vi "Format Resistor.vi"(3 "Resistor Value":dbl format="%#.3f") -> (0 "Band 2":dbl, 1 "Band 1":dbl, 2 "Band3":dbl)   [LabVIEW 2014]
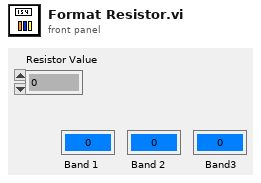
[diagram p1: front panel]
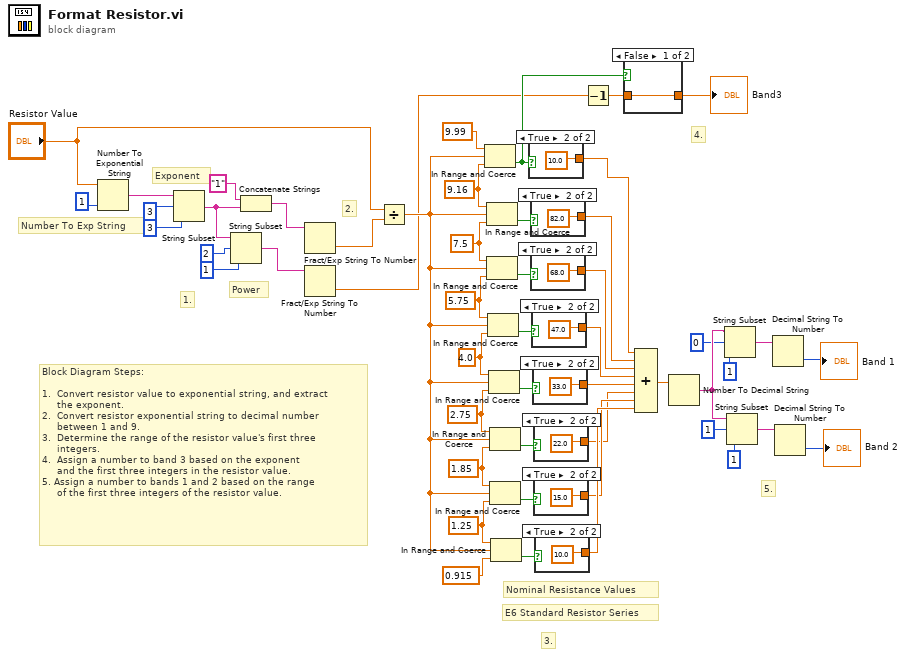
[diagram p0: block diagram]
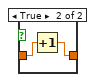
[diagram p2: hidden frame]
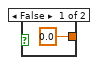
[diagram p3: hidden frame]
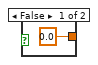
[diagram p4: hidden frame]
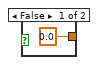
[diagram p5: hidden frame]
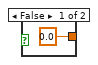
[diagram p6: hidden frame]
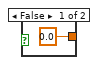
[diagram p7: hidden frame]
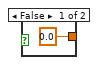
[diagram p8: hidden frame]
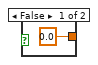
[diagram p9: hidden frame]
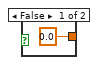
[diagram p10: hidden frame]
diagram:
  w21 = 9.16
  w27 = 7.5
  w29 = 5.75
  w26 = 4.0
  w35 = 2.75
  w34 = 1.85
  w40 = 1.25
  # "E6 Standard Resistor Series"
  # "Block Diagram Steps:\n\n1.  Convert resistor value to exponential string, and extract\n     the exponent.\n2.  Convert resistor exponential string to decimal number \n     between 1 and 9.\n3.  Determine the range of the resistor value's first three\n     integers.\n4.  Assign a number to band 3 based on the exponent\n     and the first three integers in the resistor value.\n5. Assign a number to bands 1 and 2 based on the range\n     of the first three integers of the resistor value."
  # "5."
  # "4."
  # "3."
  # "2."
  # "1."
  # "Power"
  # "Exponent"
  # "Number To Exp String"
  # "Nominal Resistance Values"
  n1 = Number To Exponential String(number="Resistor Value", precision (6)=i16 1) -> (E-format string=w49:string)  [unwired: 2 in]
  n2 = String Subset(string=w49, offset (0)=3, length (rest)=3 ("length (rest)")) -> (substring=w18:string)
  n3 = String Subset(string=w18, offset (0)=2, length (rest)=1 ("length (rest)")) -> (substring=w16:string)
  n4 = Concatenate Strings("1" ("string"), w18) -> (w45:string)
  n5 = Fract/Exp String To Number(string=w45) -> (number=w46:dbl)  [unwired: 3 in, 1 out]
  n6 = Fract/Exp String To Number(string=w16) -> (number=w12:dbl)  [unwired: 3 in, 1 out]
  n7 = Divide(x="Resistor Value", y=w46) -> (x/y=w15:dbl)
  n8 = In Range and Coerce(upper limit=9.99, x=w15, lower limit=w21) -> (In Range?=w14:bool)  [unwired: 1 out]
  n9 = In Range and Coerce(upper limit=w21, x=w15, lower limit=w27) -> (In Range?=w28:bool)  [unwired: 1 out]
  n10 = In Range and Coerce(upper limit=w27, x=w15, lower limit=w29) -> (In Range?=w30:bool)  [unwired: 1 out]
  n11 = In Range and Coerce(upper limit=w29, x=w15, lower limit=w26) -> (In Range?=w31:bool)  [unwired: 1 out]
  n12 = In Range and Coerce(upper limit=w26, x=w15, lower limit=w35) -> (In Range?=w36:bool)  [unwired: 1 out]
  n13 = In Range and Coerce(upper limit=w35, x=w15, lower limit=w34) -> (In Range?=w37:bool)  [unwired: 1 out]
  n14 = In Range and Coerce(upper limit=w34, x=w15, lower limit=w40) -> (In Range?=w41:bool)  [unwired: 1 out]
  n15 = In Range and Coerce(upper limit=w40, x=w15, lower limit=0.915) -> (In Range?=w43:bool)  [unwired: 1 out]
  n16 = case shown="True" w14 {
    tunnel: [0.0 ("lower limit") 10.0 ("lower limit")] -> w20
    frame False {
    }
    frame True {
    }
  }
  n17 = case shown="True" w28 {
    tunnel: [0.0 ("lower limit") 82.0 ("lower limit")] -> w23
    frame False {
    }
    frame True {
    }
  }
  n18 = case shown="True" w30 {
    tunnel: [0.0 ("lower limit") 68.0 ("lower limit")] -> w24
    frame False {
    }
    frame True {
    }
  }
  n19 = case shown="True" w31 {
    tunnel: [0.0 ("lower limit") 47.0 ("lower limit")] -> w25
    frame False {
    }
    frame True {
    }
  }
  n20 = case shown="True" w36 {
    tunnel: [0.0 ("lower limit") 33.0 ("lower limit")] -> w32
    frame False {
    }
    frame True {
    }
  }
  n21 = case shown="True" w37 {
    tunnel: [0.0 ("lower limit") 22.0 ("lower limit")] -> w33
    frame False {
    }
    frame True {
    }
  }
  n22 = case shown="True" w41 {
    tunnel: [0.0 ("lower limit") 15.0 ("lower limit")] -> w38
    frame False {
    }
    frame True {
    }
  }
  n23 = case shown="True" w43 {
    tunnel: [0.0 ("lower limit") 10.0 ("lower limit")] -> w39
    frame False {
    }
    frame True {
    }
  }
  n24 = Decrement(x=w12) -> (x-1=w11:dbl)
  n25 = case shown="False" w14 {
    tunnel: w11 -> [w68 w70]
    tunnel: [w68 w69] -> w13
    frame False {
    }
    frame True {
      n26 = Increment(x=w70) -> (x+1=w69:dbl)
    }
  }
  "Band3" <- w13
  n27 = Compound Arithmetic op=ADD(w20, w23, w24, w25, w32, w33, w38, w39) -> (w5:dbl)
  n28 = Number To Decimal String(number=w5) -> (decimal integer string=w10:string)  [unwired: 1 in]
  n29 = String Subset(string=w10, offset (0)=0, length (rest)=1 ("length (rest)")) -> (substring=w4:string)
  n30 = String Subset(string=w10, offset (0)=1, length (rest)=1 ("length (rest)")) -> (substring=w2:string)
  n31 = Decimal String To Number(string=w4) -> (number=→"Band 1":i32)  [unwired: 2 in, 1 out]
  n32 = Decimal String To Number(string=w2) -> (number=→"Band 2":i32)  [unwired: 2 in, 1 out]
